vi "SetCurrent.vi"(8 "error in (no error)":errorcluster, 10 "Current":T1={"area"=1, "Data"={"wl"=0.0, "power"=0.0, "voltage"=0.0, "knee"=0.0, "reverse"=0.0}} {"area" items=["CENTERA"=1, "CENTERB"=2, "CENTERC"=3, "RIGHT"=4, "TOP"=5, "LEFT"=6]}, 11 "LotData in":refnum<class "LotData.lvclass">) -> (0 "error out":errorcluster, 3 "LotData out":refnum<class "LotData.lvclass">)   [LabVIEW 2012, in "LotData.lvclass"]
uses:
  LotData.lvclass
  Controls/LotData_Current.ctl
  LotData.lvclass/LotData.ctl
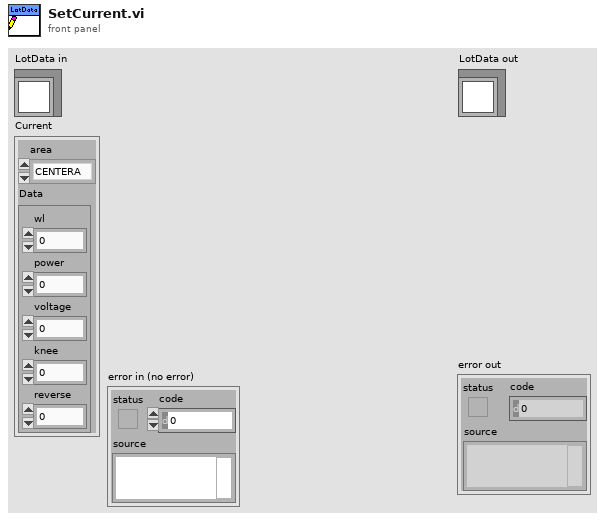
[diagram p1: front panel]
types:
  T1 = typedef "LotData.lvclass/LotData_Current.ctl" = cluster{"area":i32, "Data":cluster{"wl":dbl, "power":dbl, "voltage":dbl, "knee":dbl, "reverse":dbl}}
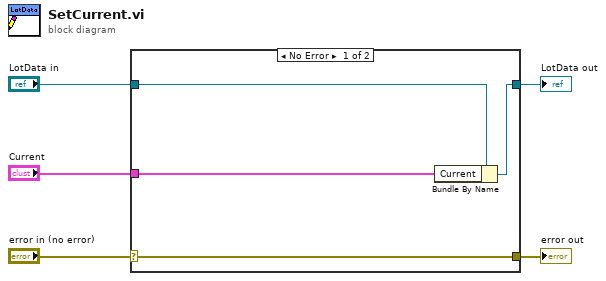
[diagram p0: block diagram]
diagram:
  n1 = case shown="No Error" "error in (no error)" {
    selector: "error in (no error)" -> [w9 w10]
    tunnel: [w9 w10] -> w4
    tunnel: [w7 w11] -> w2
    tunnel: "LotData in" -> [w8 w11]
    tunnel: "Current" -> [w6 _]
    frame No Error {
      n2 = Bundle By Name(cluster=w8, "Current"=w6) -> (w7:refnum<class "LotData.lvclass">)
    }
    frame Error {
    }
  }
  "error out" <- w4
  "LotData out" <- w2
